vi "Destroy Refs.vi"(8 "error in (no error)":errorcluster, 11 "Messaging in":refnum<class "Messaging.lvclass">) -> (0 "error out":errorcluster)   [LabVIEW 2023, in "Messaging.lvclass"]
uses:
  Messaging.lvclass
  Messaging.lvclass/Messaging.ctl
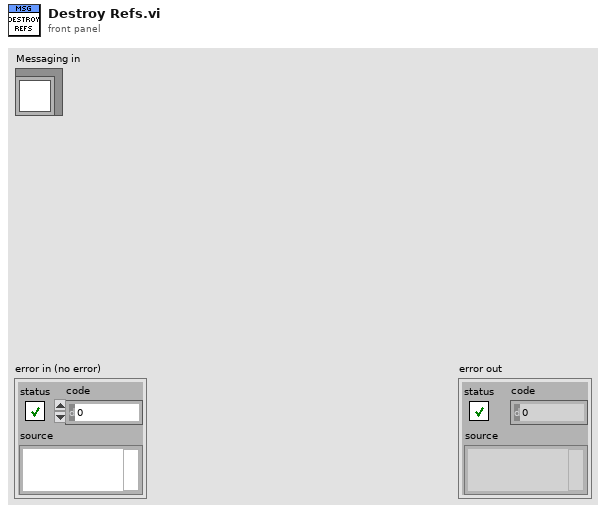
[diagram p1: front panel]
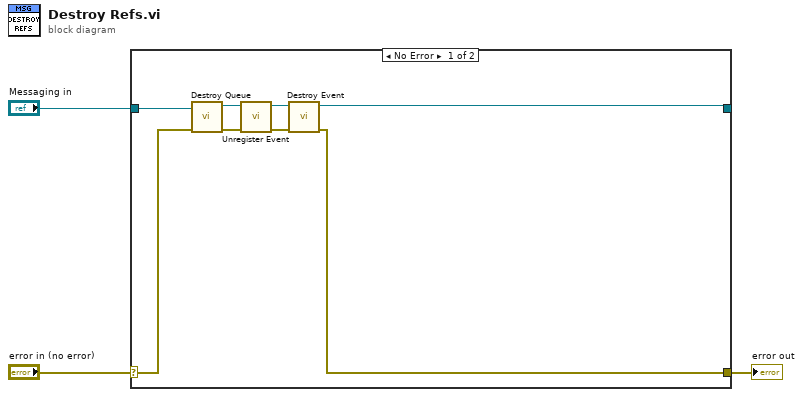
[diagram p0: block diagram]
diagram:
  n1 = case shown="No Error" "error in (no error)" {
    selector: "error in (no error)" -> [w10 w13]
    tunnel: [w5 w13] -> w2
    tunnel: [w4 w12] -> _
    tunnel: "Messaging in" -> [w11 w12]
    frame No Error {
      n2 = call "Destroy Queue.vi"("error in (no error)"=w10, "Messaging in"=w11) -> ("error out"=w9:errorcluster, "Messaging out"=w8:refnum<class "Messaging.lvclass">)  [unwired: 8 in]
      n3 = call "Unregister Event.vi"("error in (no error)"=w9, "Messaging in"=w8) -> ("error out"=w7:errorcluster, "Messaging out"=w6:refnum<class "Messaging.lvclass">)  [unwired: 8 in]
      n4 = call "Destroy Event.vi"("error in (no error)"=w7, "Messaging in"=w6) -> ("error out"=w5:errorcluster, "Messaging out"=w4:refnum<class "Messaging.lvclass">)  [unwired: 8 in]
    }
    frame Error {
    }
  }
  "error out" <- w2
